vi "configure.vi"(8 "error in (no error)":errorcluster, 11 "lv-build-default in":refnum<class "lv-builder-default.lvclass">) -> (0 "error out":errorcluster, 3 "lv-build-default out":refnum<class "lv-builder-default.lvclass">)   [LabVIEW 2015, in "lv-builder-default.lvclass"]
uses:
  lv-builder-default.lvclass
  community/_controls/command_configuration.ctl
  lv-builder-default.lvlib
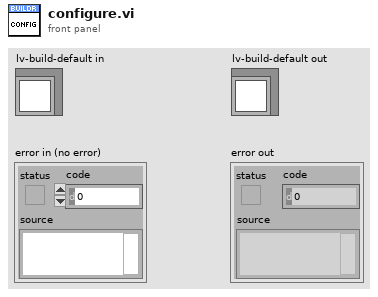
[diagram p1: front panel]
types:
  T1 = typedef "lv-builder-default.lvlib/command_configuration.ctl" = enum16{"<config_command>", "read_config", "write_config", "<null>"}
  T2 = typedef "lv-builder-default.lvlib/configuration.ctl" = cluster{"project_file":string, "lvlibp_directory":string, "zip_directory":string, "lvlib_directory":string, "update_version_vi":string, "installer_post_file":string, "distribution_folder":string, "dependencies_folder":string, "version":string, "bin_folder":string, "lvlib_post_action":u16, "installer_post_action":u16, "application_post_action":u16, "zip_post_action":u16}
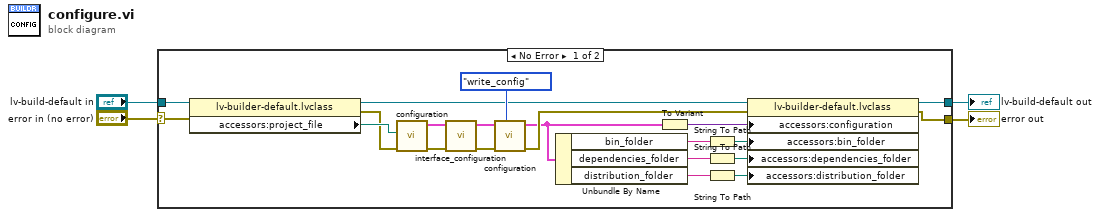
[diagram p0: block diagram]
diagram:
  n1 = case shown="No Error" "error in (no error)" {
    selector: "error in (no error)" -> [w16 w27]
    tunnel: "lv-build-default in" -> [w25 w26]
    tunnel: [w13 w27] -> w2
    tunnel: [w19 w26] -> w1
    frame No Error {
      n2 = property class="lv-builder-default.lvclass"(reference=w25, error in=w16) -> (reference out=w18:refnum<class "lv-builder-default.lvclass">, error out=w15:errorcluster, "accessors:project_file"=w17:path)
      n3 = call "configuration.vi"("error in (no error)"=w15, "project_file"=w17) -> ("error out"=w21:errorcluster, "config out"=w24:T2)  [unwired: 8 in]
      n4 = call "interface_configuration.vi"("error in (no error)"=w21, "config in"=w24) -> ("error out"=w22:errorcluster, "config out"=w23:T2)  [unwired: 8 in]
      n5 = call "configuration.vi"("command"=command_configuration."write_config", "error in (no error)"=w22, "config in"=w23) -> ("error out"=w14:errorcluster, "config out"=w11:T2)  [unwired: 7 in]
      n6 = Unbundle By Name(w11) -> ("bin_folder"=w10:string, "dependencies_folder"=w8:string, "distribution_folder"=w9:string)
      n7 = To Variant(anything=w11) -> (Variant=w12:variant)
      n8 = String To Path(string=w10) -> (path=w5:path)
      n9 = String To Path(string=w8) -> (path=w6:path)
      n10 = String To Path(string=w9) -> (path=w7:path)
      n11 = property class="lv-builder-default.lvclass"(reference=w18, error in=w14, "accessors:configuration"=w12, "accessors:bin_folder"=w5, "accessors:dependencies_folder"=w6, "accessors:distribution_folder"=w7) -> (reference out=w19:refnum<class "lv-builder-default.lvclass">, error out=w13:errorcluster)
    }
    frame Error {
    }
  }
  "error out" <- w2
  "lv-build-default out" <- w1
